vi "n x n Smoothen Array (SGL) v4.vi"(4 "Average":bool caption="Average (F)", 5 "Algorithm":T1, 6 "Threshold Low":sgl=-inf, 7 "Threshold High":sgl=inf, 8 "Error In":errorcluster, 9 "Kernel Size":i32=1, 10 "Kernel Type":T2, 11 "Array in":sgl[][](array[numeric])) -> (0 "Error Out":errorcluster, 1 "Valid?":bool[][](array[boolean]), 3 "Array out":sgl[][](array[numeric]))   [LabVIEW 2021, in "Arrays.lvlib"]
uses:
  Arrays.lvlib
  Kernel Type.ctl
  Smoothing Algorithm.ctl
  n x n Kernel Convolution (SGL).vi/d0ebc029-cbaa-4c82-a58c-923c59c440da.vi
  n x n Kernel Convolution (SGL).vi/b80d5e79-a0c8-46e2-aba9-3d60e0093a16.vi
  <vilib>/Analysis/2dsp.llb/Convolution.vi
  <vilib>/Analysis/2dsp.llb/2D Convolution (DBL).vi
  Truncate Kernel.vi
  Replace NaN by 0 (2D SGL).vi
  n x n Smoothen Array (SGL) v3.vi/d0ebc029-cbaa-4c82-a58c-923c59c440da.vi
  n x n Smoothen Array (SGL) v3.vi/b80d5e79-a0c8-46e2-aba9-3d60e0093a16.vi
  Replace NaN by 0 (2D SGL).vi/df975b44-f6c5-4554-af30-980613d33749.vi
  Compute n x n Kernel (SGL).vi
  <vilib>/Utility/error.llb/Simple Error Handler.vi
  Time/Time.lvlib
panel:
  out "elapsed (relative) seconds":dbl
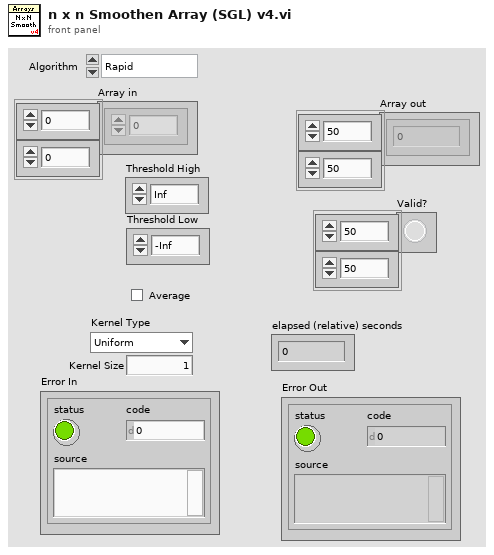
[diagram p1: front panel]
types:
  T1 = typedef "Arrays.lvlib/Smoothing Algorithm.ctl" = enum16{"Rapid", "Thorough"}
  T2 = typedef "Arrays.lvlib/Kernel Type.ctl" = enum16{"Uniform", "Bilinear", "Gaussian"}
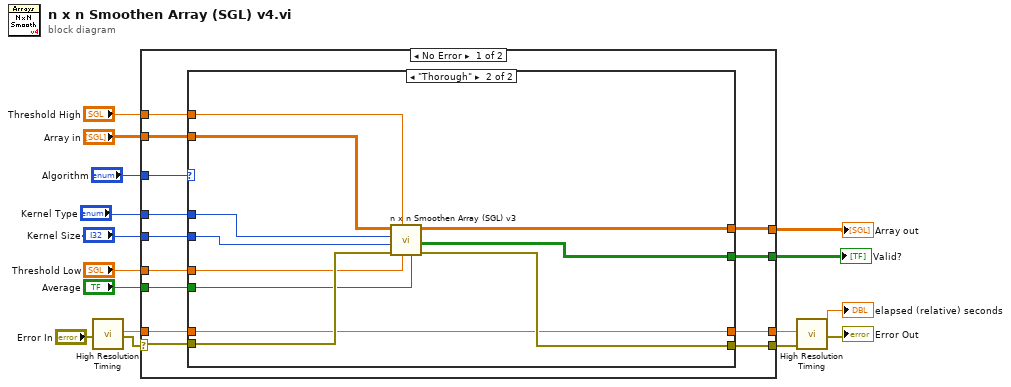
[diagram p0: block diagram]
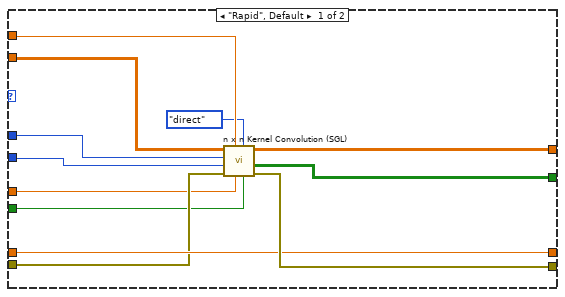
[diagram p2: hidden frame]
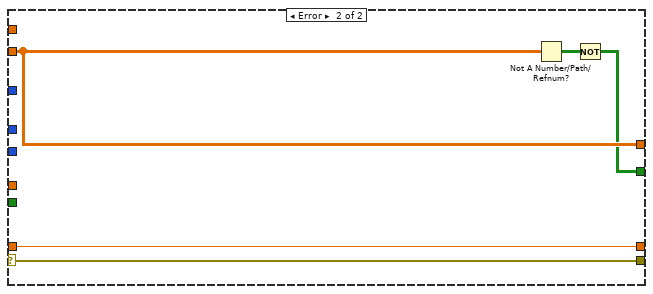
[diagram p3: hidden frame]
diagram:
  n1 = call "High Resolution Timing.vi"("Error In"="Error In") -> ("elapsed (relative) seconds"=w5:dbl, "Error Out"=w6:errorcluster)  [unwired: 16 in, 1 out]
  n2 = case shown="No Error" w6 {
    selector: w6 -> [w24 w53]
    tunnel: "Array in" -> [w28 w56]
    tunnel: "Kernel Size" -> [w26 _]
    tunnel: [w20 w56] -> w15
    tunnel: "Threshold Low" -> [w22 _]
    tunnel: "Threshold High" -> [w27 _]
    tunnel: [w19 w55] -> w14
    tunnel: [w17 w54] -> w3
    tunnel: "Kernel Type" -> [w25 _]
    tunnel: "Average" -> [w21 _]
    tunnel: w5 -> [w18 w54]
    tunnel: [w23 w53] -> w2
    tunnel: "Algorithm" -> [w29 _]
    frame No Error {
      n3 = case shown="\"Thorough\"" w29 {
        tunnel: w28 -> [w41 w52]
        tunnel: w27 -> [w33 w51]
        tunnel: w26 -> [w35 w49]
        tunnel: w25 -> [w34 w50]
        tunnel: w24 -> [w36 w48]
        tunnel: [w38 w47] -> w23
        tunnel: w22 -> [w32 w46]
        tunnel: w21 -> [w31 w45]
        tunnel: [w40 w44] -> w20
        tunnel: [w39 w43] -> w19
        tunnel: w18 -> [w37 w42]
        tunnel: [w37 w42] -> w17
        frame "Rapid", Default {
          n4 = call "n x n Kernel Convolution (SGL).vi"("Average"=w31, "Convolution Algorithm (direct)"=enum32{"direct", "frequency domain"}."direct", "Threshold Low"=w32, "Threshold High"=w33, "Error In"=w36, "Kernel Size"=w35, "Kernel Type"=w34, "Array in"=w41) -> ("Error Out"=w38:errorcluster, "Valid?"=w39:bool[][], "Array out"=w40:sgl[][])  [unwired: 1 in]
        }
        frame "Thorough" {
          n5 = call "n x n Smoothen Array (SGL) v3.vi"("Average"=w45, "Threshold Low"=w46, "Threshold High"=w51, "Error In"=w48, "Kernel Size"=w49, "Kernel Type"=w50, "Array in"=w52) -> ("Error Out"=w47:errorcluster, "Valid?"=w43:bool[][], "Array out"=w44:sgl[][])  [unwired: 2 in]
        }
      }
    }
    frame Error {
      n6 = Not A Number/Path/Refnum?(number/path/refnum=w56) -> (NaN/Path/Refnum?=w57:bool[][])
      n7 = Not(x=w57) -> (.not. x?=w55:bool[][])
    }
  }
  "Array out" <- w15
  "Valid?" <- w14
  n8 = call "High Resolution Timing.vi"("relative seconds (NaN)"=w3, "Error In"=w2) -> ("elapsed (relative) seconds"=→"elapsed (relative) seconds":dbl, "Error Out"=→"Error Out":errorcluster)  [unwired: 15 in, 1 out]
